vi "Read Engine Alarms.vi"(0 "class data in":refnum<class "MB_ENGINE.lvclass">, 11 "error in (no error)":errorcluster) -> (4 "class data out":refnum<class "MB_ENGINE.lvclass">, 6 "Alarms":T1, 15 "error out":errorcluster)   [LabVIEW 2019, in "MB_ENGINE.lvclass"]
uses:
  MB_ENGINE.lvclass
  Engine Alarms.ctl
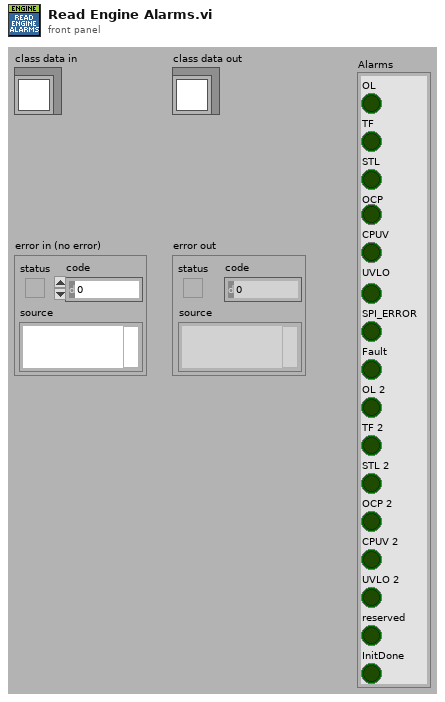
[diagram p1: front panel]
types:
  T1 = typedef "MB_ENGINE.lvclass/Engine Alarms.ctl" = cluster{"OL":bool, "TF":bool, "STL":bool, "OCP":bool, "CPUV":bool, "UVLO":bool, "SPI_ERROR":bool, "Fault":bool, "OL 2":bool, "TF 2":bool, "STL 2":bool, "OCP 2":bool, "CPUV 2":bool, "UVLO 2":bool, "reserved":bool, "InitDone":bool}
  T2 = cluster{"Boolean array[0]":bool, "Boolean array[1]":bool, "Boolean array[2]":bool, "Boolean array[3]":bool, "Boolean array[4]":bool, "Boolean array[5]":bool, "Boolean array[6]":bool, "Boolean array[7]":bool, "Boolean array[8]":bool, "Boolean array[9]":bool, "Boolean array[10]":bool, "Boolean array[11]":bool, "Boolean array[12]":bool, "Boolean array[13]":bool, "Boolean array[14]":bool, "Boolean array[15]":bool}
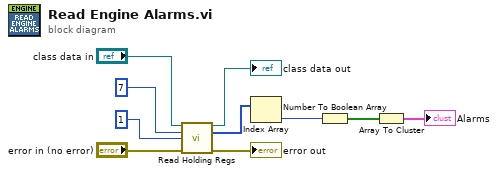
[diagram p0: block diagram]
diagram:
  n1 = call-dynamic "Read Holding Regs.vi"("reference in"="class data in", "starting address"=u16 7, "number of inputs"=u16 1, "error in (no error)"="error in (no error)") -> ("reference out"=→"class data out":refnum<class "MB_ENGINE.lvclass">, "register values"=w2:u16[], "error out"=→"error out":errorcluster)  [unwired: 9 in]
  n2 = Index Array(array=w2) -> (element=w5:u16)  [unwired: 1 in]
  n3 = Number To Boolean Array(number=w5) -> (Boolean array=w4:bool[])
  n4 = Array To Cluster(array=w4) -> (cluster=→"Alarms":T2)
